vi "Read Modules.vi"(8 "error in (no error)":errorcluster, 11 "ModuleAbstract in":refnum<class "ModuleAbstract.lvclass">) -> (0 "error out":errorcluster, 2 "Modules":T1, 3 "ModuleAbstract out":refnum<class "ModuleAbstract.lvclass">)   [LabVIEW 2019, in "ModuleAbstract.lvlib" / "ModuleAbstract.lvclass"]
uses:
  ModuleAbstract.lvclass
  Containers/ActorRefContainer/TypeDef/Active Modules REF.ctl
  <vilib>/ActorFramework/Message Enqueuer/Message Enqueuer.lvclass
  ModuleAbstract.lvclass/ModuleAbstract.ctl
  Containers/ActorRefContainer/ActorRefContainer.lvclass/ActorRefContainer.ctl
  Containers/ActorRefContainer/ActorRefContainer.lvclass
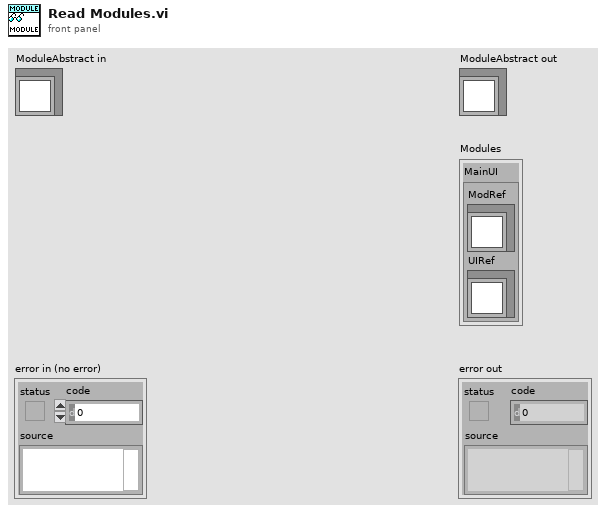
[diagram p1: front panel]
types:
  T1 = typedef "ActorRefContainer.lvlib/ActorRefContainer.lvclass/Active Modules REF.ctl" = cluster{"MainUI":cluster{"ModRef":refnum<class "Message Enqueuer.lvclass">, "UIRef":refnum<class "Message Enqueuer.lvclass">}}
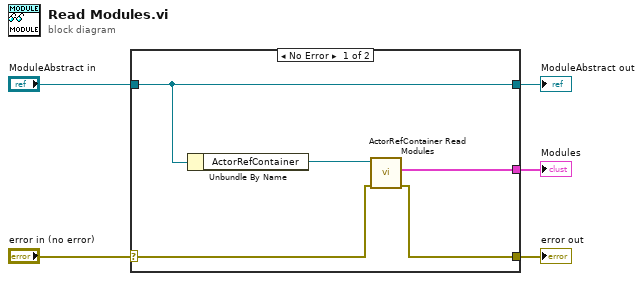
[diagram p0: block diagram]
diagram:
  n1 = case shown="No Error" "error in (no error)" {
    selector: "error in (no error)" -> [w7 w11]
    tunnel: [w6 w11] -> w4
    tunnel: [w10 w12] -> w2
    tunnel: "ModuleAbstract in" -> [w10 w12]
    tunnel: [w8 _] -> w1
    frame No Error {
      n2 = Unbundle By Name(w10) -> ("ActorRefContainer"=w9:refnum<class "ActorRefContainer.lvclass">)
      n3 = call "ActorRefContainer Read Modules.vi"("error in (no error)"=w7, "ActorRefContainer in"=w9) -> ("error out"=w6:errorcluster, "Modules"=w8:T1)  [unwired: 7 in, 1 out]
    }
    frame Error {
    }
  }
  "error out" <- w4
  "ModuleAbstract out" <- w2
  "Modules" <- w1
